vi "Grabber Angles to Position.vi"(8 "Forerm Length":dbl, 9 "Backarm Length":dbl, 10 "Forearm Angle Degrees":dbl, 11 "Backarm Angle Degrees":dbl) -> (2 "Y Final":dbl, 3 "X Final":dbl)   [LabVIEW 2017]
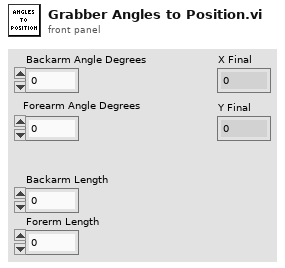
[diagram p1: front panel]
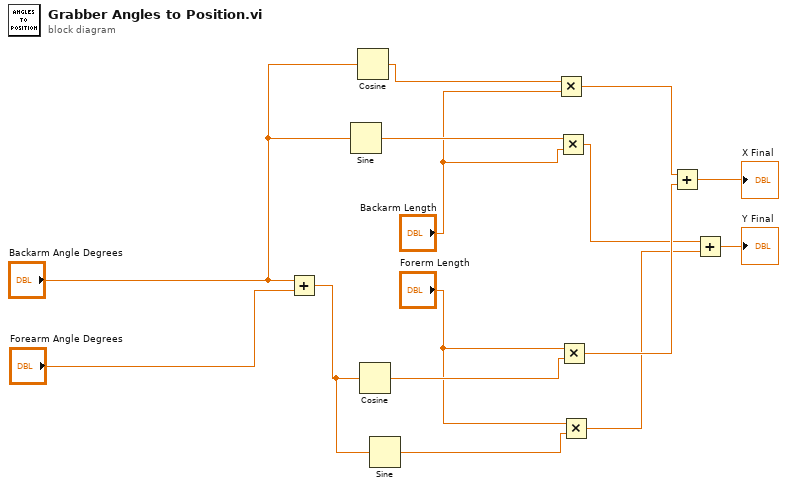
[diagram p0: block diagram]
diagram:
  n1 = Add(x="Backarm Angle Degrees", y="Forearm Angle Degrees") -> (x+y=w15:dbl)
  n2 = Sine(x="Backarm Angle Degrees") -> (sin(x)=w13:dbl)
  n3 = Cosine(x="Backarm Angle Degrees") -> (cos(x)=w14:dbl)
  n4 = Cosine(x=w15) -> (cos(x)=w11:dbl)
  n5 = Sine(x=w15) -> (sin(x)=w9:dbl)
  n6 = Multiply(x=w14, y="Backarm Length") -> (x*y=w8:dbl)
  n7 = Multiply(x=w13, y="Backarm Length") -> (x*y=w5:dbl)
  n8 = Multiply(x="Forerm Length", y=w11) -> (x*y=w7:dbl)
  n9 = Multiply(x="Forerm Length", y=w9) -> (x*y=w3:dbl)
  n10 = Add(x=w8, y=w7) -> (x+y=→"X Final":dbl)
  n11 = Add(x=w5, y=w3) -> (x+y=→"Y Final":dbl)
